vi "Get Count.vi"(8 "error in (no error)":errorcluster, 11 "Test Actor API":refnum<class "Test Actor API.lvclass">) -> (0 "error out":errorcluster, 3 "Count":i32)   [LabVIEW 2020, in "Test Actor API.lvclass"]
uses:
  Test Actor API.lvclass
  C:/dev/PGS/2001 - TBCM/Source/RT/RTAF/Source/RTAF/Actors/Base Actor/API/Actor API.lvclass
  Base Actor/API/Actor API.lvclass
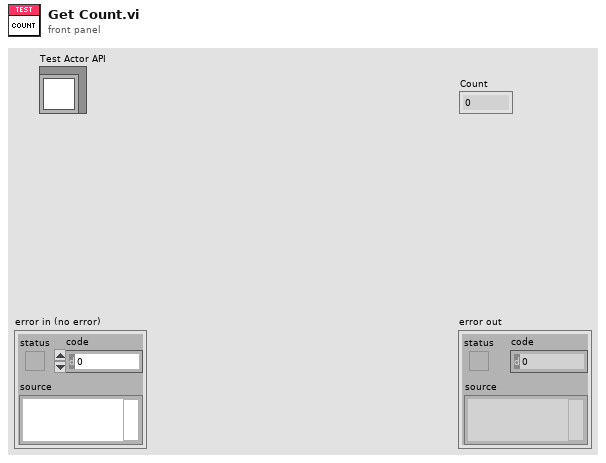
[diagram p1: front panel]
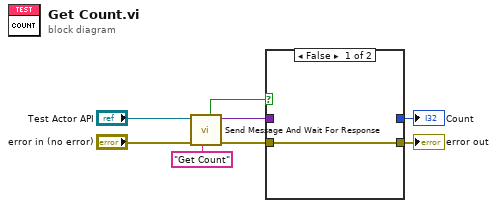
[diagram p0: block diagram]
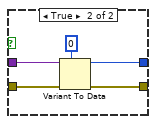
[diagram p2: hidden frame]
diagram:
  n1 = call "Send Message And Wait For Response.vi"("Name"="Get Count", "error in (no error)"="error in (no error)", "Actor API in"="Test Actor API") -> ("error out"=w5:errorcluster, "Response"=w3:variant, "Response Received"=w4:bool)  [unwired: 6 in]
  n2 = case shown="False" w4 {
    tunnel: w5 -> [w9 w13]
    tunnel: w3 -> [_ w14]
    tunnel: [_ w11] -> w2
    tunnel: [w9 w10] -> w1
    frame False {
    }
    frame True {
      n3 = Variant To Data(error in=w13, type=0, Variant=w14) -> (data=w11:i32, error out=w10:errorcluster)
    }
  }
  "error out" <- w1
  "Count" <- w2
